vi "Create MsgQ.vi"(8 "error in (no error)":errorcluster) -> (0 "error out":errorcluster)   [LabVIEW 2013, in "Main MsgQ.lvlib"]
doc: "Creates a message queue for each item in the enumerated type:\nShecduler User Interface, Scheduler TCP/IP, Stacker send, Scanner Send\nQueues have same name as enum"
uses:
  Main MsgQ.lvlib
  Common/Interloop MessageQ/Message que instance modes enum.ctl
  Common/Interloop MessageQ/Interloop MessageQ.lvlib
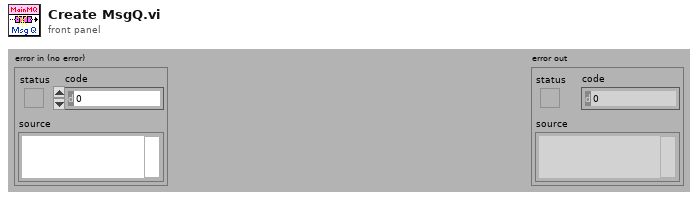
[diagram p1: front panel]
types:
  T1 = typedef "Interloop MessageQ.lvlib/Message que instance modes enum.ctl" = enum16{"Initialize", "Broadcast Message", "Send Message", "Read Message", "Kill"}
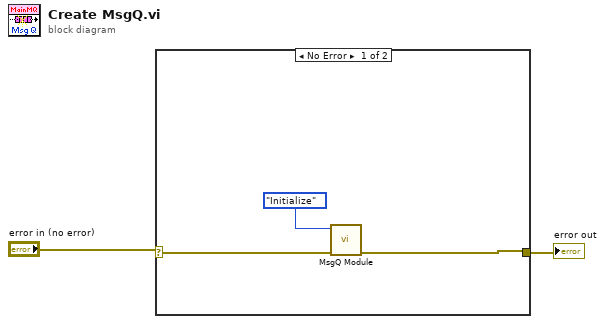
[diagram p0: block diagram]
diagram:
  n1 = case shown="No Error" "error in (no error)" {
    selector: "error in (no error)" -> [w4 w6]
    tunnel: [w3 w6] -> w1
    frame No Error {
      n2 = call "MsgQ Module.vi"("error in (no error)"=w4, "Mode"=Message_que_instance_modes_enum."Initialize") -> ("error out"=w3:errorcluster)  [unwired: 6 in, 3 out]
    }
    frame Error {
    }
  }
  "error out" <- w1
